vi "Set Hardware Relay State.vi"(0 "PhysicalChannelRelay in":refnum<class "PhysicalChannelRelay.lvclass">, 5 "session in":refnum<k21>, 7 "device in":refnum<k21>, 9 "RelayAction":T1=21 items=["CloseRelay"=21, "OpenRelay"=20], 11 "error in (no error)":errorcluster) -> (4 "PhysicalChannelRelay out":refnum<class "PhysicalChannelRelay.lvclass">, 6 "session out":refnum<k21>, 8 "device out":refnum<k21>, 15 "error out":errorcluster)   [LabVIEW 2015, in "PhysicalChannelRelay.lvclass"]
doc: "This uses a device physical channel to set the current hardware state of a relay."
uses:
  PhysicalChannelRelay.lvclass
  slscsl/RelayAction.ctl
  Relay Interface/Commit Buffer Action.ctl
  PhysicalChannelRelay.lvclass/PhysicalChannelRelay.ctl
  <vilib>/SLSC/Set Phys Chan Property (Bool).vi
  Relay Interface/RelayInterface.lvclass
  <vilib>/SLSC/SLSC.lvlib
  slscsl/slscsl.lvclass
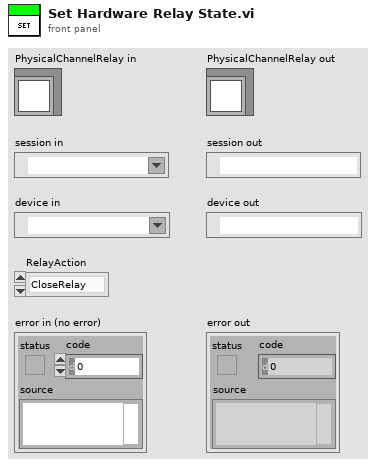
[diagram p1: front panel]
types:
  T1 = typedef "slscsl.lvclass/RelayAction.ctl" = u32
  T2 = typedef "RelayInterface.lvclass/Commit Buffer Action.ctl" = enum16{"Get Session Buffer", "Add Transaction", "Clear Session Buffer", "Clear All"}
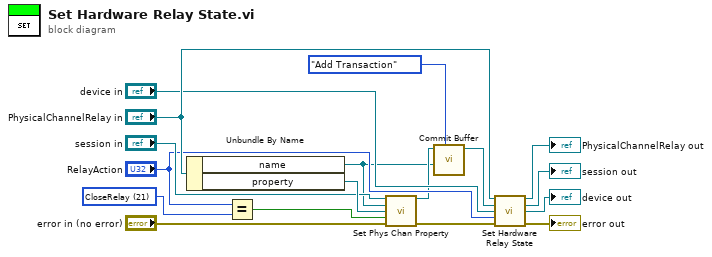
[diagram p0: block diagram]
diagram:
  w6 = T1 21 items=["CloseRelay"=21, "OpenRelay"=20] ("RelayAction")
  n1 = Unbundle By Name("PhysicalChannelRelay in") -> ("name"=w1:refnum<k21>, "property"=w16:refnum<k21>)
  n2 = Equal?(x="RelayAction", y=w6) -> (x = y?=w17:bool)
  n3 = call-poly <vilib>:"Set Phys Chan Property.vi"("session in"="session in", "physical channels"=w1, "property"=w16, "property value"=w17, "error in (no error)"="error in (no error)") -> ("session out"=w4:refnum<k21>, "error out"=w5:errorcluster)  [unwired: 9 in]
  n4 = call "Commit Buffer.vi"("Action"=Commit_Buffer_Action."Add Transaction", "Transation String"=w1, "session in"=w4) -> ("session out"=w3:refnum<k21>)  [unwired: 7 in, 1 out]
  n5 = call-parent "Set Hardware Relay State.vi"("RelayInterface in"="PhysicalChannelRelay in", "session in"=w3, "device in"="device in", "relay action (Close Relay)"="RelayAction", "error in (no error)"=w5) -> ("RelayInterface out"=→"PhysicalChannelRelay out":refnum<class "PhysicalChannelRelay.lvclass">, "session out"=→"session out":refnum<k21>, "device out"=→"device out":refnum<k21>, "error out"=→"error out":errorcluster)  [unwired: 7 in]
